vi "run_embedding_core.vi"(0 "llm_openai_embedding in":refnum<class "llm_gemini_embedding.lvclass">, 5 "data":refnum<class "abstract_message_base.lvclass">[](array[class]), 11 "error in (no error)":errorcluster) -> (4 "llm_openai_embedding out":refnum<class "llm_gemini_embedding.lvclass">, 6 "embedding response":refnum<class "message_vectors.lvclass">[](array[class]), 15 "error out":errorcluster)   [LabVIEW 2020, in "llm_gemini_embedding.lvclass"]
uses:
  llm_gemini_embedding.lvclass
  abstract_message_base/abstract_message_base.lvclass
  message_vectors/message_vectors.lvclass
  <vilib>/httpClient/POSTBuffer.vi
  <vilib>/httpClient/LabVIEWHTTPClient.lvlib
panel:
  out "body":string
  out "headers":string
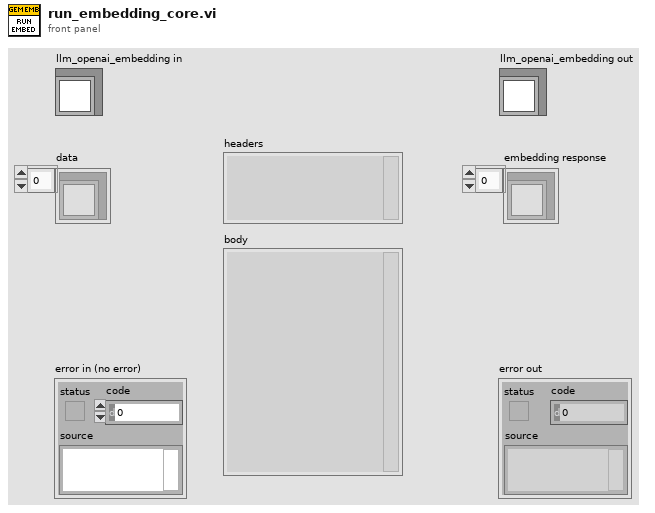
[diagram p1: front panel]
types:
  T1 = typedef "llm_gemini_embedding.lvclass/request_Data.ctl" = cluster{"model":string, "content":cluster{"parts":cluster{"text":string}[]}}
  T2 = typedef "LabVIEWHTTPClient.lvlib/ClientHandle.ctl" = refnum<k1>
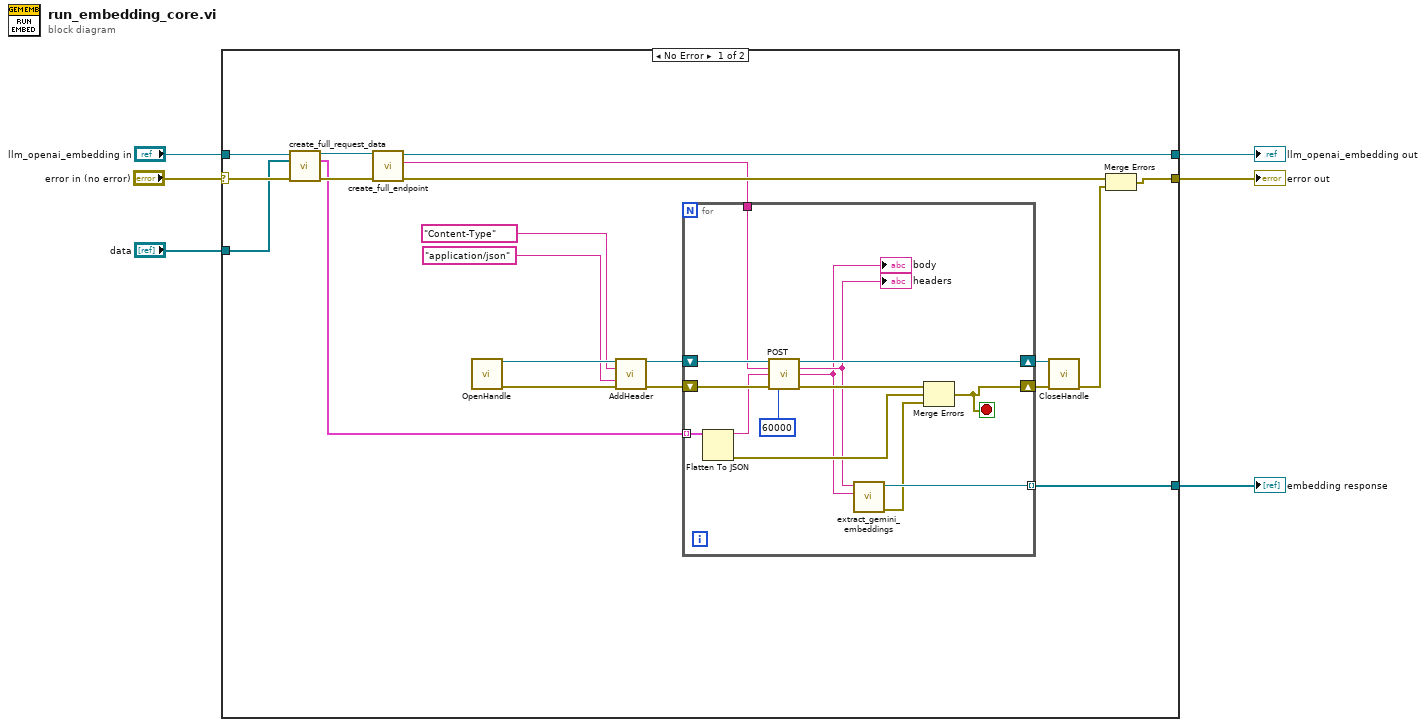
[diagram p0: block diagram]
diagram:
  n1 = case shown="No Error" "error in (no error)" {
    selector: "error in (no error)" -> [w13 w42]
    tunnel: [w10 w42] -> w5
    tunnel: [w19 w41] -> w4
    tunnel: "llm_openai_embedding in" -> [w14 w41]
    tunnel: "data" -> [w12 _]
    tunnel: [w8 _] -> w1
    frame No Error {
      n2 = call-dynamic "create_full_request_data.vi"("llm_openai_embedding in"=w14, "data"=w12, "error in (no error)"=w13) -> ("llm_openai_embedding out"=w15:refnum<class "llm_gemini_embedding.lvclass">, "request_data"=w7:T1[], "error out"=w16:errorcluster)  [unwired: 10 in]
      n3 = call-dynamic "create_full_endpoint.vi"("error in (no error)"=w16, "llm_openai_embedding in"=w15) -> ("error out"=w18:errorcluster, "endpoint"=w17:string, "llm_openai_embedding out"=w19:refnum<class "llm_gemini_embedding.lvclass">)  [unwired: 7 in]
      n4 = call <vilib>:"OpenHandle.vi"() -> ("client handle out"=w26:T2, "error out"=w25:errorcluster)  [unwired: 14 in]
      n5 = call <vilib>:"AddHeader.vi"("client handle"=w26, "header"="Content-Type", "value"="application/json", "error in (no error)"=w25) -> ("client handle out"=w22:T2, "error out"=w21:errorcluster)  [unwired: 10 in]
      n6 = for {
        tunnel: w17 -> [w36]
        shift-right: [w38] -> w20
        shift-left: w22 -> [w40]
        tunnel: w7 -> [w34] mode=indexing
        shift-right: [w31] -> w11
        shift-left: w21 -> [w39]
        tunnel: [w28] -> w8 mode=indexing
        stop <- w31 stop-if-true
        n7 = Flatten To JSON(anything=w34) -> (JSON string=w33:string, 11:w32:errorcluster)  [unwired: 2 in]
        n8 = call-poly <vilib>:"POST.vi"("client handle"=w40, "url"=w36, "buffer"=w33, "error in (no error)"=w39, "timeout (10000)"=60000) -> ("client handle out"=w38:T2, "headers"=w30:string, "body"=w29:string, "error out"=w35:errorcluster)  [unwired: 7 in]
        "headers" <- w30
        "body" <- w29
        n9 = call "extract_gemini_embeddings.vi"("body"=w29, "headers"=w30) -> ("error out"=w27:errorcluster, "vector response"=w28:refnum<class "message_vectors.lvclass">)  [unwired: 8 in]
        n10 = Merge Errors(w35, w32, w27) -> (w31:errorcluster)
      }
      n11 = call <vilib>:"CloseHandle.vi"("client handle"=w20, "error in (no error)"=w11) -> ("error out"=w9:errorcluster)  [unwired: 13 in]
      n12 = Merge Errors(w18, w9) -> (w10:errorcluster)
    }
    frame Error {
    }
  }
  "error out" <- w5
  "llm_openai_embedding out" <- w4
  "embedding response" <- w1
